vi "Get TreeIndex from ID.vi"(8 "error in (no error)":errorcluster, 11 "Node ID":string) -> (0 "error out":errorcluster, 3 "TreeIndex":i32)   [LabVIEW 2015, in "Configuration Tool.lvlib"]
uses:
  Configuration Tool.lvlib
  <vilib>/NI/Configuration Framework/Node/NISE_CEF_Node.lvclass/NISE_CEF_Node.ctl
  <vilib>/NI/Configuration Framework/Node/ReadParent.vi
  <vilib>/NI/Configuration Framework/Node/ReadChildren.vi
  <vilib>/NI/Configuration Framework/Node/NISE_CEF_Node.lvclass
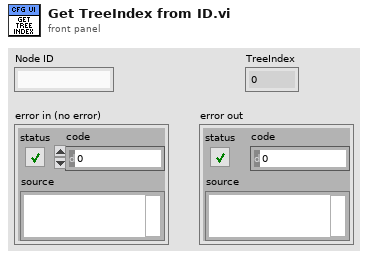
[diagram p1: front panel]
types:
  T1 = typedef "NISE_CEF_Node.lvclass/NodeRef.ctl" = refnum<data-value>
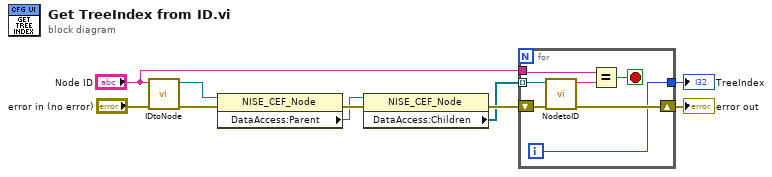
[diagram p0: block diagram]
diagram:
  n1 = call <vilib>:"IDtoNode.vi"("error in"="error in (no error)", "ID"="Node ID") -> ("error out"=w10:errorcluster, "node ref"=w7:T1)  [unwired: 7 in, 1 out]
  n2 = property on="Property Node" class="NISE_CEF_Node"(reference=w7, error in=w10) -> (error out=w8:errorcluster, "DataAccess:Parent"=w4:T1)  [unwired: 1 out]
  n3 = property class="NISE_CEF_Node"(reference=w4, error in=w8) -> (error out=w5:errorcluster, "DataAccess:Children"=w3:T1[])  [unwired: 1 out]
  n4 = for {
    shift-right: [w17] -> w6
    shift-left: w5 -> [w15]
    tunnel: w3 -> [w14] mode=indexing
    tunnel: "Node ID" -> [w13]
    tunnel: [w11] -> w1
    i -> [w11]
    stop <- w12 stop-if-true
    n5 = call <vilib>:"NodetoID.vi"("error in"=w15, "node ref"=w14) -> ("error out"=w17:errorcluster, "ID"=w16:string)  [unwired: 8 in]
    n6 = Equal?(x=w13, y=w16) -> (x = y?=w12:bool)
  }
  "error out" <- w6
  "TreeIndex" <- w1
